vi "HapticBumpForce.vi"(0 "Target Position [deg]":dbl, 1 "Haptic Bump Force [N]":dbl, 3 "Position [deg]":dbl, 5 "Are we within haptic bump range?":bool=TRUE, 7 "Plateau length":dbl, 9 "Ramp length":dbl) -> (19 "CurrentOut [A]":dbl)   [LabVIEW 2019]
panel:
  out "In Ramp Range?":bool
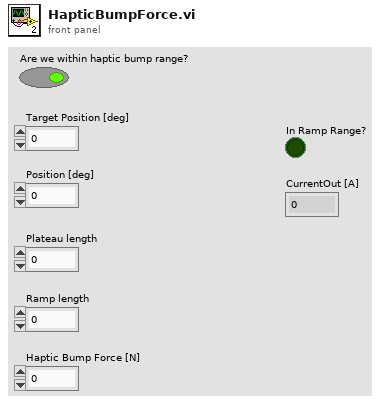
[diagram p1: front panel]
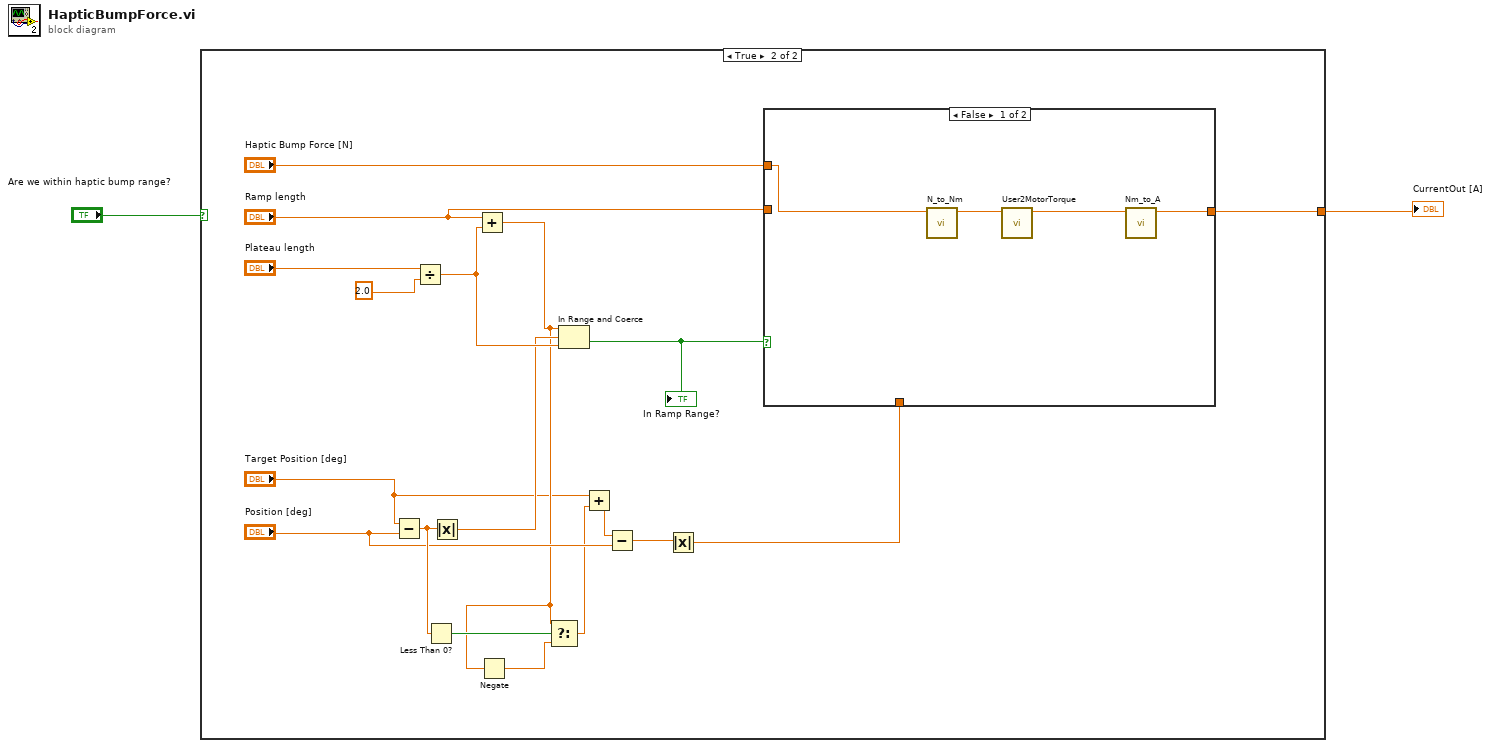
[diagram p0: block diagram]
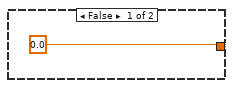
[diagram p2: hidden frame]
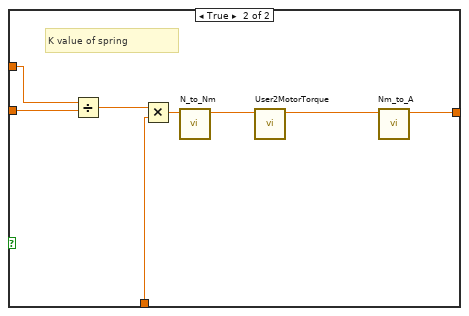
[diagram p3: hidden frame]
diagram:
  n1 = case shown="True" "Are we within haptic bump range?" {
    tunnel: [0.0 w4] -> w1
    frame False {
    }
    frame True {
      n2 = Subtract(x="Target Position [deg]", y="Position [deg]") -> (x-y=w16:dbl)
      n3 = Divide(x="Plateau length", y=2.0) -> (x/y=w18:dbl)
      n4 = Less Than 0?(x=w16) -> (x < 0?=w15:bool)
      n5 = Absolute Value(x=w16) -> (abs(x)=w17:dbl)
      n6 = Add(x="Ramp length", y=w18) -> (x+y=w10:dbl)
      n7 = Negate(x=w10) -> (-x=w9:dbl)
      n8 = Select(t=w10, s=w15, f=w9) -> (s? t:f=w8:dbl)
      n9 = In Range and Coerce(upper limit=w10, x=w17, lower limit=w18) -> (In Range?=w21:bool)  [unwired: 1 out]
      "In Ramp Range?" <- w21
      n10 = Add(x="Target Position [deg]", y=w8) -> (x+y=w14:dbl)
      n11 = Subtract(x=w14, y="Position [deg]") -> (x-y=w12:dbl)
      n12 = Absolute Value(x=w12) -> (abs(x)=w11:dbl)
      n13 = case shown="False" w21 {
        tunnel: [w23 w30] -> w4
        tunnel: w11 -> [_ w29]
        tunnel: "Ramp length" -> [_ w26]
        tunnel: "Haptic Bump Force [N]" -> [w22 w27]
        frame False {
          n14 = call "N_to_Nm.vi"("Force [N]"=w22) -> ("Torque [Nm]"=w25:dbl)  [unwired: 10 in]
          n15 = call "User2MotorTorque.vi"("User Torque [Nm]"=w25) -> ("Motor Torque [Nm]"=w24:dbl)  [unwired: 10 in]
          n16 = call "Nm_to_A.vi"("Torque [Nm]"=w24) -> ("Current [A]"=w23:dbl)  [unwired: 10 in]
        }
        frame True {
          # "K value of spring"
          n17 = Divide(x=w27, y=w26) -> (x/y=w28:dbl)
          n18 = Multiply(x=w28, y=w29) -> (x*y=w32:dbl)
          n19 = call "N_to_Nm.vi"("Force [N]"=w32) -> ("Torque [Nm]"=w33:dbl)  [unwired: 10 in]
          n20 = call "User2MotorTorque.vi"("User Torque [Nm]"=w33) -> ("Motor Torque [Nm]"=w31:dbl)  [unwired: 10 in]
          n21 = call "Nm_to_A.vi"("Torque [Nm]"=w31) -> ("Current [A]"=w30:dbl)  [unwired: 10 in]
        }
      }
    }
  }
  "CurrentOut [A]" <- w1
